vi "ConcatenateOntoShortcutMenu.vi"(8 "error in":errorcluster, 9 "menu ref in":refnum<k9>, 11 "Abstract Engine":refnum<class "Abstract Engine.lvclass">) -> (0 "error out":errorcluster, 1 "menu ref out":refnum<k9>, 3 "Abstract Engine out":refnum<class "Abstract Engine.lvclass">)   [LabVIEW 2025, in "Abstract Engine.lvlib" / "Abstract Engine.lvclass"]
doc: "Allows children to insert menu items without overriding ShortcutMenu.vi entirely. By default, called after Add/Remove.Copyright 2017 National Instruments Corporation\n\nLicensed under the Apache License, Version 2.0 (the \"License\"); you may not use this file except in compliance with the License. You may obtain a copy of the License at http://www.apache.org/licenses/LICENSE-2.0\nUnless required by applicable law or agreed to in writing, software distributed under the License is distributed on an \"AS IS\" BASIS, WITHOUT WARRANTIES OR CONDITIONS OF ANY KIND, either express or implied. See the License for the specific language governing permissions and limitations under the License."
uses:
  Abstract Engine.lvclass
  Abstract Engine.lvclass/Abstract Engine.ctl
  Read Initialized.vi
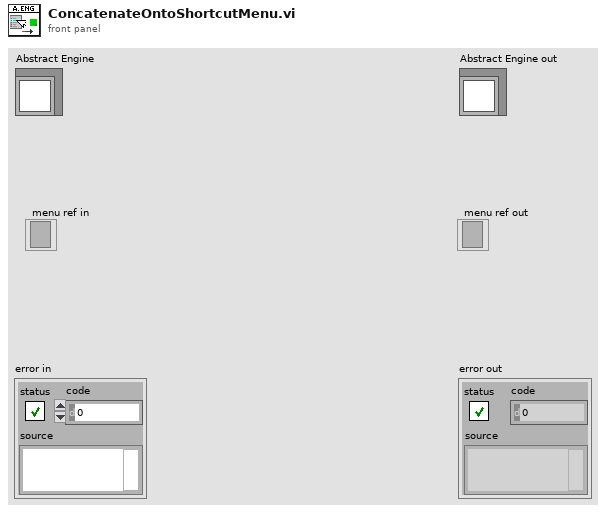
[diagram p1: front panel]
types:
  T1 = typedef "Abstract Engine.lvlib/Abstract Engine.lvclass/Engine Cluster.ctl" = cluster{"IP Address":string, "Type":string, "Initialized":bool, "InstrumentMap":map{string, cluster{"Initialized":bool, "Channels":T2[]}}}
  T2 = typedef "Abstract Engine.lvlib/Abstract Instrument.lvclass/Channel.ctl" = cluster{"Alias":string, "Type":enum16{"Numeric", "Boolean", "String"}, "Unit":T3, "Upper limit":dbl, "Lower limit":dbl, "Measurement":variant}
  T3 = typedef "Abstract Engine.lvlib/Abstract Instrument.lvclass/Unit.ctl" = enum16{"---", "V", "A", "Ohm", "Hz", "uF", "degC", "deg"}
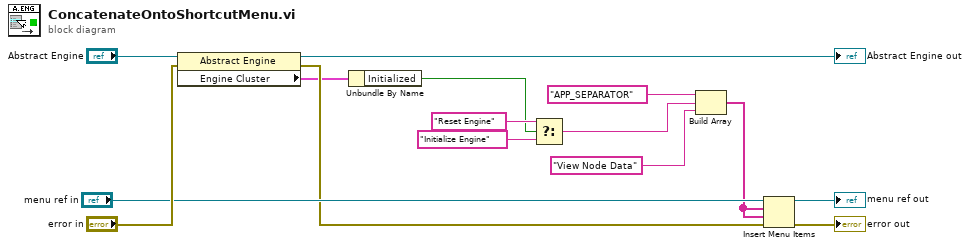
[diagram p0: block diagram]
diagram:
  n1 = property class="Abstract Engine"(reference="Abstract Engine", error in="error in") -> (reference out=→"Abstract Engine out":refnum<class "Abstract Engine.lvclass">, error out=w11:errorcluster, "Engine Cluster"=w2:T1)
  n2 = Unbundle By Name(w2) -> ("Initialized"=w1:bool)
  n3 = Select(t="Reset Engine", s=w1, f="Initialize Engine") -> (s? t:f=w5:string)
  n4 = Build Array("APP_SEPARATOR", w5, "View Node Data") -> (w4:string[])
  n5 = Insert Menu Items(6:w11, 7:w4, 8:w4, 9:"menu ref in") -> (0:→"error out":errorcluster, 3:→"menu ref out":refnum<k9>)  [unwired: 2 in, 1 out]
